vi "Draw Floor.vi"(8 "error in (no error)":errorcluster, 11 "name":string="Floor") -> (0 "error out":errorcluster, 3 "floor object":refnum<vi>)   [LabVIEW 2015]
doc: "Creates the 3D floor object."
uses:
  <vilib>/Utility/miscctls.llb/LV3DPointTypeDef.ctl
  <vilib>/Utility/miscctls.llb/LVTextureCoordinateArrayTypeDef.ctl
  <vilib>/picture/3D Picture Control/Object/Create Object (name).vi
  <vilib>/picture/3D Picture Control/NI_3D Picture Control.lvlib
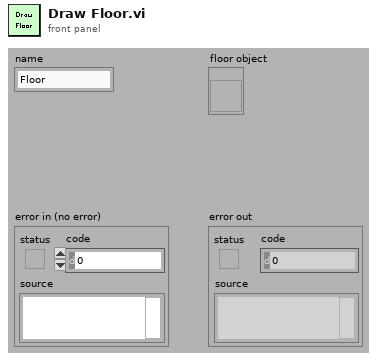
[diagram p1: front panel]
types:
  T1 = typedef "LVTextureCoordinateArrayTypeDef.ctl" = cluster{"S":sgl, "T":sgl}[]
  T2 = typedef "LV3DPointTypeDef.ctl" = cluster{"X":sgl, "Y":sgl, "Z":sgl}
  T3 = enum16{"Overall", "Per Primitive", "Per Vertex", "Binding Off"}
  T4 = enum16{"Points", "Lines", "Line Strip", "Line Loop", "Triangles", "Triangle Strip", "Triangle Fan", "Quads", "Quad Strip", "Polygon"}
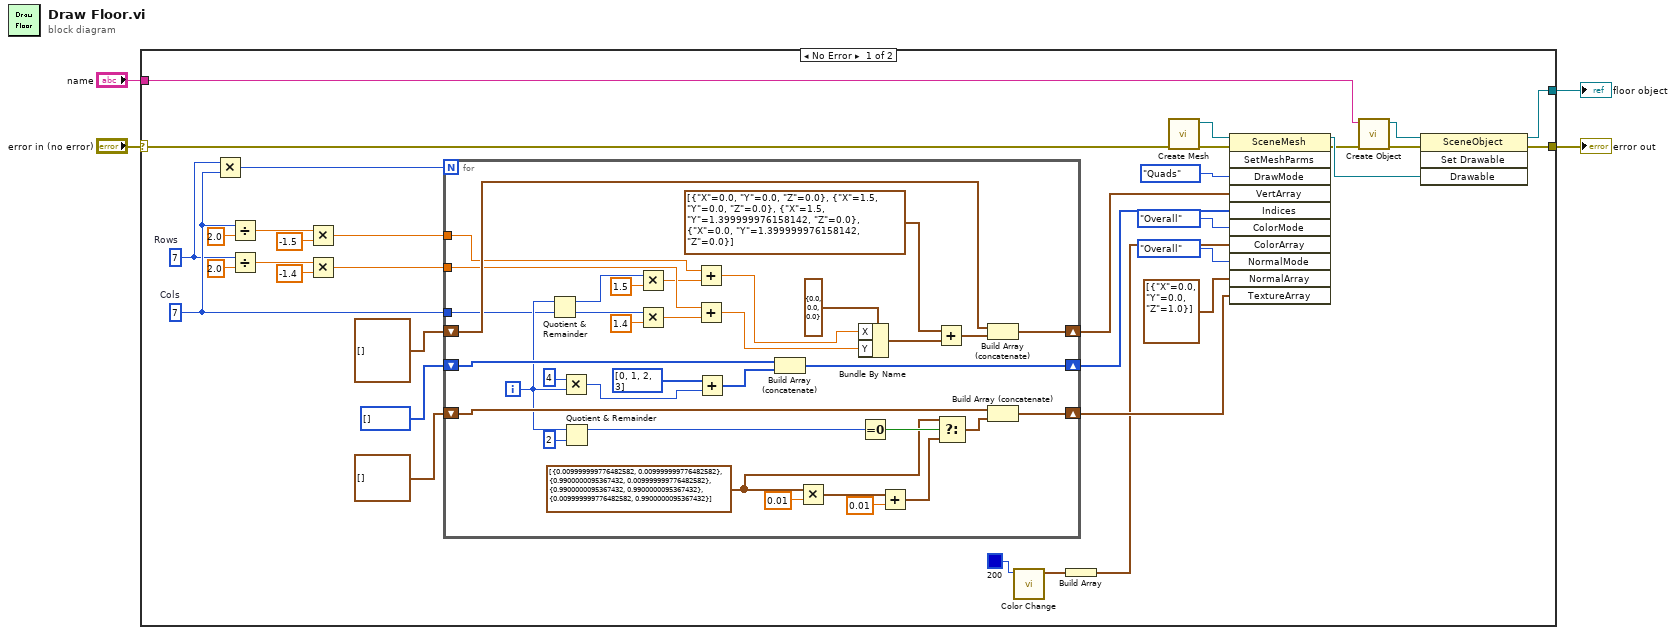
[diagram p0: block diagram]
diagram:
  n1 = case shown="No Error" "error in (no error)" {
    selector: "error in (no error)" -> [w8 w74]
    tunnel: "name" -> [w14 _]
    tunnel: [w10 _] -> w3
    tunnel: [w9 w74] -> w2
    frame No Error {
      w38 = 7  # Cols
      w29 = 7  # Rows
      n2 = Multiply(x=w29, y=w38) -> (x*y=w28:i32)
      n3 = Divide(x=w38, y=2.0 ("x/y")) -> (x/y=w34:dbl)
      n4 = Divide(x=w29, y=2.0 ("x/y")) -> (x/y=w32:dbl)
      n5 = Multiply(x=w34, y=-1.5) -> (x*y=w37:dbl)
      n6 = Multiply(x=w32, y=-1.4) -> (x*y=w36:dbl)
      n7 = for {
        N: w28 -> [_]
        shift-right: [w73] -> w26
        shift-left: u32[] [] -> [w72]
        shift-right: [w71] -> w27
        shift-left: T2[] [] -> [w70]
        shift-right: [w68] -> w25
        shift-left: T1 [] ("Texture Coordinate Array") -> [w69]
        tunnel: w36 -> [w50]
        tunnel: w37 -> [w44]
        tunnel: w38 -> [w51]
        i -> [w52]
        w58 = T1 [{"S"=0.01, "T"=0.01}, {"S"=0.99, "T"=0.01}, {"S"=0.99, "T"=0.99}, {"S"=0.01, "T"=0.99}] ("Texture Coordinate Array")
        n8 = Quotient & Remainder(x=w52, y=w51) -> (x-y*floor(x/y)=w43:i32, floor(x/y)=w48:i32)
        n9 = Multiply(x=4, y=w52) -> (x*y=w64:i32)
        n10 = Quotient & Remainder(x=w52, y=2) -> (x-y*floor(x/y)=w60:i32)  [unwired: 1 out]
        n11 = Multiply(x=w43, y=1.5) -> (x*y=w45:dbl)
        n12 = Multiply(x=w48, y=1.4) -> (x*y=w49:dbl)
        n13 = Add(x=w44, y=w45) -> (x+y=w41:dbl)
        n14 = Add(x=w50, y=w49) -> (x+y=w40:dbl)
        n15 = Add(x=u32[] [0, 1, 2, 3] ("Indices"), y=w64) -> (x+y=w62:u32[])
        n16 = Build Array (concatenate)(w72, w62) -> (w73:u32[])
        n17 = Multiply(x=w58, y=0.01 ("T")) -> (x*y=w55:cluster{"S":dbl, "T":dbl}[])
        n18 = Bundle By Name(cluster=T2 {"X"=0.0, "Y"=0.0, "Z"=0.0} ("3D Point"), "X"=w41, "Y"=w40) -> (w39:T2)
        n19 = Equal To 0?(x=w60) -> (x = 0?=w59:bool)
        n20 = Add(x=w55, y=0.01 ("T")) -> (x+y=w53:cluster{"S":dbl, "T":dbl}[])
        n21 = Add(x=T2[] [{"X"=0.0, "Y"=0.0, "Z"=0.0}, {"X"=1.5, "Y"=0.0, "Z"=0.0}, {"X"=1.5, "Y"=1.4, "Z"=0.0}, {"X"=0.0, "Y"=1.4, "Z"=0.0}] ("Vertex Array"), y=w39) -> (x+y=w66:T2[])
        n22 = Select(t=w58, s=w59, f=w53) -> (s? t:f=w56:cluster{"S":dbl, "T":dbl}[])
        n23 = Build Array (concatenate)(w70, w66) -> (w71:T2[])
        n24 = Build Array (concatenate)(w69, w56) -> (w68:cluster{"S":dbl, "T":dbl}[])
      }
      n25 = call <vilib>:"Color Change.vi"("Color"=u32 200) -> ("RGBA"=w20:cluster{"R":sgl, "G":sgl, "B":sgl, "A":sgl})  [unwired: 1 in, 9 out]
      n26 = Build Array(w20) -> (w21:cluster{"R":sgl, "G":sgl, "B":sgl, "A":sgl}[])
      n27 = call <vilib>:"Create Mesh.vi"("error in (no error)"=w8) -> ("error out"=w7:errorcluster, "New Mesh Refnum"=w11:refnum<vi>)  [unwired: 9 out]
      n28 = invoke class="SceneMesh" method="SetMeshParms"(reference=w11, error in=w7, "DrawMode"=T4."Quads" ("Draw Mode"), "VertArray"=w27, "Indices"=w26, "ColorMode"=T3."Overall" ("Color Binding Mode"), "ColorArray"=w21, "NormalMode"=T3."Overall" ("Normal Binding Mode"), "NormalArray"=T2[] [{"X"=0.0, "Y"=0.0, "Z"=1.0}] ("Normal Array"), "TextureArray"=w25) -> (reference out=w16:refnum<vi>, error out=w6:errorcluster)  [unwired: 1 in, 9 out]
      n29 = call-poly <vilib>:"Create Object.vi"("error in (no error)"=w6, "Name"=w14) -> ("error out"=w5:errorcluster, "Scene:New Object"=w15:refnum<vi>)  [unwired: 8 in]
      n30 = invoke class="SceneObject" method="Set Drawable"(reference=w15, error in=w5, "Drawable"=w16) -> (reference out=w10:refnum<vi>, error out=w9:errorcluster)  [unwired: 1 in, 2 out]
    }
    frame Error {
    }
  }
  "floor object" <- w3
  "error out" <- w2
